vi "fromXml.vi"(8 "error in (no error)":errorcluster, 10 "dataPointXml":refnum<class "xmlNode.lvclass">, 11 "ScriptEvent in":refnum<class "ScriptEvent.lvclass">) -> (0 "error out":errorcluster, 3 "ScriptEvent out":refnum<class "ScriptEvent.lvclass">)   [LabVIEW 2009, in "Tools.lvlib" / "Scripting.lvlib" / "ScriptEvent.lvclass"]
uses:
  ScriptEvent.lvclass
  xmlNode/xmlNode.lvclass
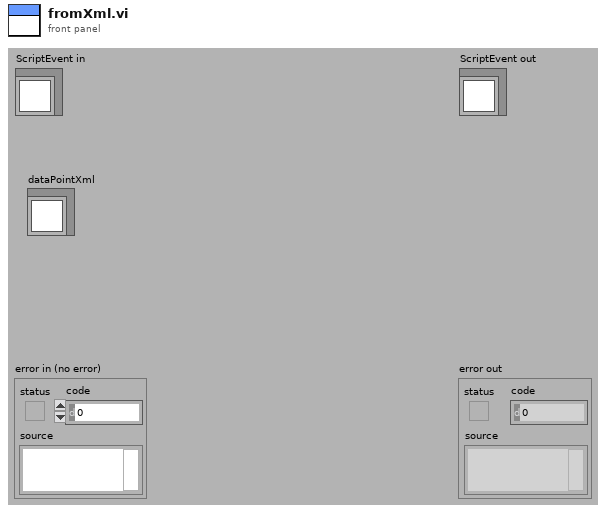
[diagram p1: front panel]
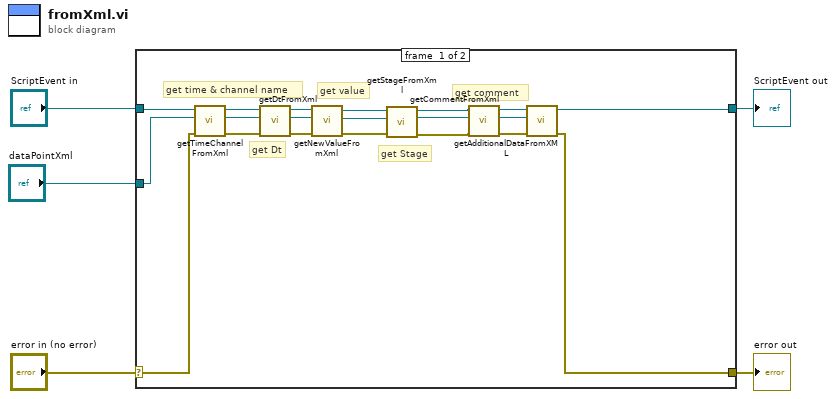
[diagram p0: block diagram]
diagram:
  n1 = case shown="No Error" "error in (no error)" {
    selector: "error in (no error)" -> [w23 w27]
    tunnel: [w7 w27] -> w4
    tunnel: [w6 w26] -> w2
    tunnel: "ScriptEvent in" -> [w25 w26]
    tunnel: "dataPointXml" -> [w24 _]
    frame #0 {
      # "get comment"
      # "get Stage"
      # "get value"
      # "get Dt"
      # "get time & channel name"
      n2 = call "getTimeChannelFromXml.vi"("error in (no error)"=w23, "Xml"=w24, "ScriptEvent in"=w25) -> ("error out"=w20:errorcluster, "Xml"=w21:refnum<class "xmlNode.lvclass">, "ScriptEvent out"=w22:refnum<class "ScriptEvent.lvclass">)  [unwired: 6 in]
      n3 = call "getDtFromXml.vi"("error in (no error)"=w20, "Xml"=w21, "ScriptEvent in"=w22) -> ("error out"=w17:errorcluster, "Xml out"=w18:refnum<class "xmlNode.lvclass">, "ScriptEvent out"=w19:refnum<class "ScriptEvent.lvclass">)  [unwired: 6 in]
      n4 = call-dynamic "getNewValueFromXml.vi"("error in (no error)"=w17, "Xml"=w18, "ScriptEvent in"=w19) -> ("error out"=w15:errorcluster, "Xml out"=w14:refnum<class "xmlNode.lvclass">, "ScriptEvent out"=w16:refnum<class "ScriptEvent.lvclass">)  [unwired: 6 in]
      n5 = call "getStageFromXml.vi"("error in (no error)"=w15, "Xml"=w14, "ScriptEvent in"=w16) -> ("error out"=w11:errorcluster, "Xml out"=w12:refnum<class "xmlNode.lvclass">, "ScriptEvent out"=w13:refnum<class "ScriptEvent.lvclass">)  [unwired: 6 in]
      n6 = call "getCommentFromXml.vi"("error in (no error)"=w11, "Xml"=w12, "ScriptEvent in"=w13) -> ("error out"=w8:errorcluster, "Xml out"=w9:refnum<class "xmlNode.lvclass">, "ScriptEvent out"=w10:refnum<class "ScriptEvent.lvclass">)  [unwired: 6 in]
      n7 = call-dynamic "getAdditionalDataFromXML.vi"("error in (no error)"=w8, "Xml"=w9, "ScriptEvent in"=w10) -> ("error out"=w7:errorcluster, "ScriptEvent out"=w6:refnum<class "ScriptEvent.lvclass">)  [unwired: 6 in, 1 out]
    }
    frame #1 {
    }
  }
  "error out" <- w4
  "ScriptEvent out" <- w2
